vi "Find Messages Folders.vi"(8 "错误输入（无错误）":errorcluster, 11 "项目输入":refnum<vi>) -> (0 "错误输出":errorcluster, 3 "Messages Folders":map{string, refnum<vi>}(c390))   [LabVIEW 2020]
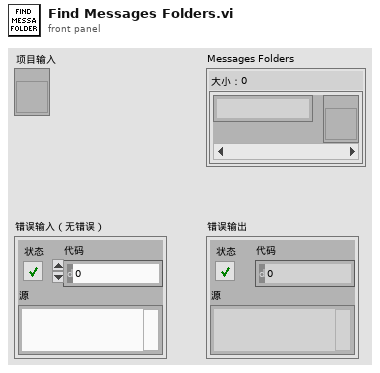
[diagram p1: front panel]
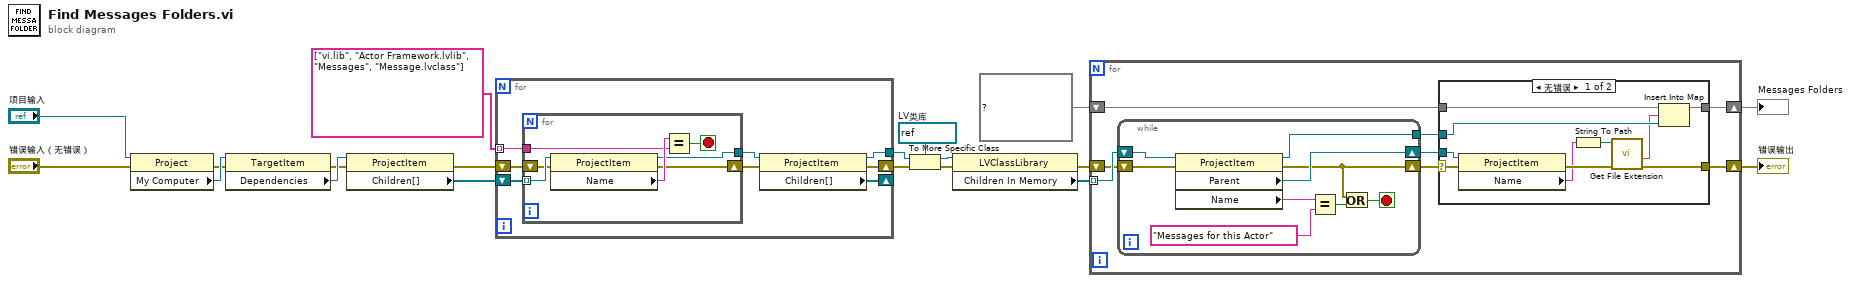
[diagram p0: block diagram]
diagram:
  w15 = refnum<vi> refnum  # LV类库
  n1 = property class="Project"(reference="项目输入", error in="错误输入（无错误）") -> (error out=w7:errorcluster, "My Computer"=w13:refnum<vi>)  [unwired: 1 out]
  n2 = property class="TargetItem"(reference=w13, error in=w7) -> (error out=w6:errorcluster, "Dependencies"=w12:refnum<vi>)  [unwired: 1 out]
  n3 = property class="ProjectItem"(reference=w12, error in=w6) -> (error out=w5:errorcluster, "Children[]"=w11:refnum<vi>[])  [unwired: 1 out]
  n4 = for {
    shift-right: [w25] -> _
    shift-left: w11 -> [w27]
    tunnel: string[] ["vi.lib", "Actor Framework.lvlib", "Messages", "Message.lvclass"] -> [w24] mode=indexing
    tunnel: [w23] -> w10
    shift-right: [w20] -> w4
    shift-left: w5 -> [w22]
    n5 = for {
      tunnel: w27 -> [w34] mode=indexing
      tunnel: [w31] -> w26
      tunnel: w24 -> [w30]
      shift-right: [w28] -> w21
      shift-left: w22 -> [w29]
      stop <- w32 stop-if-true
      n6 = property class="ProjectItem"(reference=w34, error in=w29) -> (reference out=w31:refnum<vi>, error out=w28:errorcluster, "Name"=w33:string)
      n7 = Equal?(x=w33, y=w30) -> (x = y?=w32:bool)
    }
    n8 = property class="ProjectItem"(reference=w26, error in=w21) -> (reference out=w23:refnum<vi>, error out=w20:errorcluster, "Children[]"=w25:refnum<vi>[])
  }
  n9 = To More Specific Class(target class=w15, reference=w10, error in=w4) -> (specific class reference=w9:refnum<vi>, error out=w3:errorcluster)
  n10 = property class="LVClassLibrary"(reference=w9, error in=w3) -> (error out=w2:errorcluster, "Children In Memory"=w8:refnum<vi>[])  [unwired: 1 out]
  n11 = for {
    tunnel: w8 -> [w38] mode=indexing
    shift-right: [w39] -> w19
    shift-left: w2 -> [w37]
    shift-right: [w41] -> w17
    shift-left: map{string, refnum<vi>} {} ("映射表") -> [w42]
    n12 = while {
      shift-right: [w50] -> w40
      shift-left: w38 -> [w51]
      tunnel: [w47] -> w35
      shift-right: [w43] -> w36
      shift-left: w37 -> [w46]
      stop <- w45 stop-if-true
      n13 = property class="ProjectItem"(reference=w51, error in=w46) -> (reference out=w47:refnum<vi>, error out=w43:errorcluster, "Parent"=w50:refnum<vi>, "Name"=w48:string)
      n14 = Equal?(x=w48, y="Messages for this Actor") -> (x = y?=w44:bool)
      n15 = Or(x=w43, y=w44) -> (x .or. y?=w45:bool)
    }
    n16 = case shown="无错误" w36 {
      selector: w36 -> [w57 _]
      tunnel: w35 -> [w59 _]
      tunnel: w42 -> [w61 w62]
      tunnel: [w60 w62] -> w41
      tunnel: w40 -> [w58 _]
      tunnel: [w55 _] -> w39
      frame No Error {
        n17 = property class="ProjectItem"(reference=w58, error in=w57) -> (error out=w54:errorcluster, "Name"=w53:string)  [unwired: 1 out]
        n18 = String To Path(string=w53) -> (path=w56:path)
        n19 = call <vilib>:"Get File Extension.vi"("error in (no error)"=w54, "file"=w56) -> ("error out"=w55:errorcluster, "filename without extension"=w52:string)  [unwired: 5 in, 3 out]
        n20 = Insert Into Map(map in=w61, key=w52, value=w59) -> (map out=w60:map{string, refnum<vi>})  [unwired: 2 out]
      }
      frame Error {
      }
    }
  }
  "错误输出" <- w19
  "Messages Folders" <- w17
